vi "CTR_StartOutputFreqs.vi"(7 "DeviceIndex":u32, 8 "error in (no error)":errorcluster, 10 "WriteClockHz":dbl, 11 "ReadClockHz":dbl) -> (0 "error out":errorcluster, 2 "Actual WriteClockHz":dbl, 3 "Actual ReadClockHz":dbl)   [LabVIEW 2012]
doc: "unsigned long CTR_StartOutputFreq(\nunsigned long DeviceIndex - number from 0-31 indicating on which device you wish to output a\nfrequency\nunsigned long BlockIndex - number indicating which 8254 you wish to output a frequency from\ndouble *pHz - pointer to a double precision IEEE floating point number containing the desired\noutput frequency. This value is set by the driver to the actual frequency that will be output, as\nlimited by the device’s capabilities.\n)\nCTR_8254SelectGate() and CTR_8254ReadLatched() are used in measuring frequency. To\nmeasure frequency one must count pulses for a known duration. In simplest terms, the number of\npulses that occur for 1 second translates directly to Hertz. In the USB-CTR-15 and other\nsupported devices, you can create a known duration by configuring one counter to act as a\n“gating” signal for any collection of other counters. The other “measurement” counters will only\ncount during the “high” side of the gate signal, which we can control.\nSo, to measure frequency you 1) create a gate signal of known duration; 2) connect this gating\nsignal to the gate pins of all the “measurement” counters; 3) call CTR_8254SelectGate() to tell\nthe board which counter is generating that gate; and 4) call CTR_8254ReadLatched()\nperiodically to read the latched count values from all the “measurement” counters.\nIn practice, it may not be possible to generate a gating signal of sufficient duration from a single\ncounter. Simply concatenate two or more counters into a series, or daisy-chain, and use the last\ncounter’s output as your gating signal. This last counter in the chain should be reported as the\n“gate source” using CTR_8254SelectGate().\nOnce a value has been read from a counter using the CTR_8254ReadLatched() call, it can be\ntranslated into actual Hz by dividing the count value returned by the high-side-duration of the\ngating signal, in seconds. For example, if your gate is configured for 10Hz, the high-side lasts\n0.05seconds; if you read 1324 counts"
uses:
  Windows/System32/AIOUSB.dll
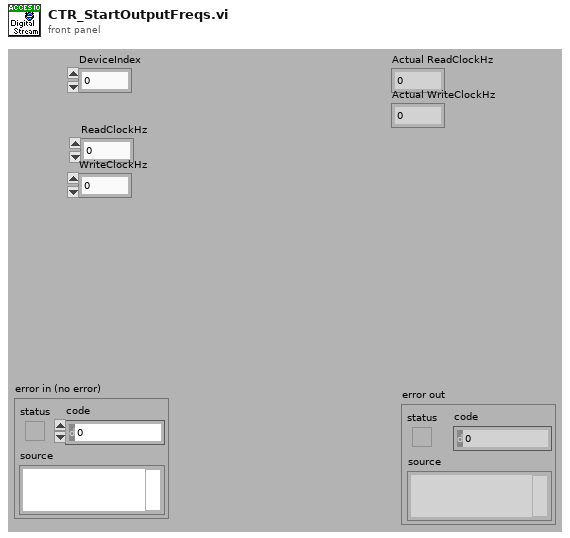
[diagram p1: front panel]
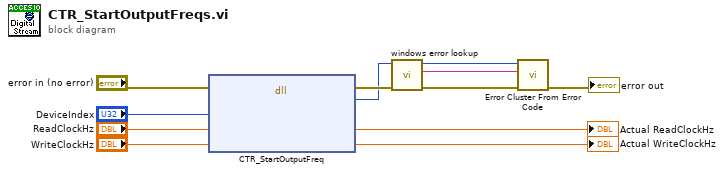
[diagram p0: block diagram]
diagram:
  n1 = dll-call lib="C:/Windows/System32/AIOUSB.dll" fn="CTR_StartOutputFreq"(error in="error in (no error)", "DeviceIndex"="DeviceIndex", "ReadClockHz"="ReadClockHz", "WriteClockHz"="WriteClockHz") -> (error out=w8:errorcluster, "return type"=w7:u32, "ReadClockHz"=→"Actual ReadClockHz":dbl, "WriteClockHz"=→"Actual WriteClockHz":dbl)  [unwired: 3 in, 1 out]
  n2 = call "windows error lookup.vi"("error in (no error)"=w8, "Error Code"=w7) -> ("error out"=w10:errorcluster, "error message (\"\")"=w11:string)  [unwired: 8 in]
  n3 = call <vilib>:"Error Cluster From Error Code.vi"("error in (no error)"=w10, "error message (\"\")"=w11, "error code (0)"=w7) -> ("error out"=→"error out":errorcluster)  [unwired: 6 in]
